vi "sine_gen.vi"(5 "prev_val":u32, 6 "reset_accum":bool, 7 "phase_shift 2":u32, 8 "frequency":u32=100, 9 "sine_amp":dbl=10.0 format="%#_13g", 10 "step_time(ms)":u32) -> (0 "next_val":u32, 3 "sine_out":dbl)   [LabVIEW 2018]
panel:
  out "freq_increment_1":u32=429496730
  out "sine_out_plot":dbl(graph)=-8.272652363658558
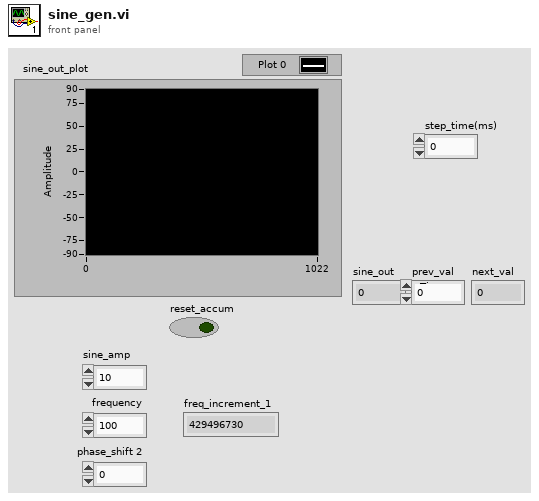
[diagram p1: front panel]
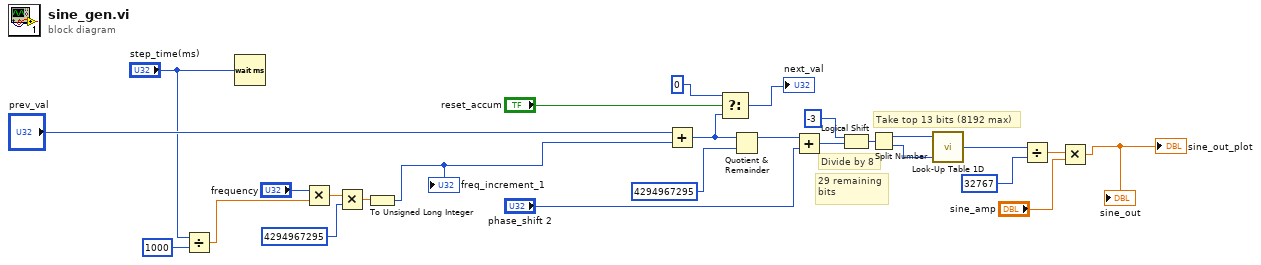
[diagram p0: block diagram]
diagram:
  # "Take top 13 bits (8192 max)"
  # "29 remaining\nbits"
  # "Divide by 8"
  n1 = Divide(x="step_time(ms)", y=u32 1000) -> (x/y=w2:dbl)
  n2 = Wait (ms)(milliseconds to wait="step_time(ms)") -> ()  [unwired: 1 out]
  n3 = Multiply(x="frequency", y=w2) -> (x*y=w8:dbl)
  n4 = Multiply(x=w8, y=u32 4294967295) -> (x*y=w9:dbl)
  n5 = To Unsigned Long Integer(number=w9) -> (unsigned 32bit integer=w11:u32)
  "freq_increment_1" <- w11
  n6 = Add(x="prev_val", y=w11) -> (x+y=w18:u32)
  n7 = Select(t=u32 0, s="reset_accum", f=w18) -> (s? t:f=→"next_val":u32)
  n8 = Quotient & Remainder(x=w18, y=u32 4294967295) -> (x-y*floor(x/y)=w24:u32)  [unwired: 1 out]
  n9 = Add(x=w24, y="phase_shift 2") -> (x+y=w23:u32)
  n10 = Logical Shift(y=i16 -3, x=w23) -> (x << y=w21:u32)
  n11 = Split Number(x=w21) -> (hi(x)=w20:u16, lo(x)=w19:u16)
  n12 = call "Look-Up Table 1D"("address"=w20, "fractional index (x 2^16)"=w19) -> ("data out"=w15:i16)  [unwired: 7 in]
  n13 = Divide(x=w15, y=i16 32767) -> (x/y=w13:dbl)
  n14 = Multiply(x=w13, y="sine_amp") -> (x*y=→"sine_out_plot" →"sine_out":dbl)
